vi "Add New XML Tag.vi"(5 "Tag Data":string, 7 "Tag Name":string, 8 "error in (no error)":errorcluster, 10 "Owning Element":refnum<k20>, 11 "XML File Ref in":refnum<k20>) -> (0 "error out":errorcluster, 2 "dup Owning Element":refnum<k20>, 3 "XML File Ref out":refnum<k20>)   [LabVIEW 2020, in "LVLIBP CD XML Updater.lvlib" / "Project XML Editor.lvclass"]
uses:
  Project XML Editor.lvclass
  <vilib>/xml/Close Reference(Node).vi
  <resource>/objmgr/DOMUserDefRef.rc
  <vilib>/xml/NI_XML.lvlib
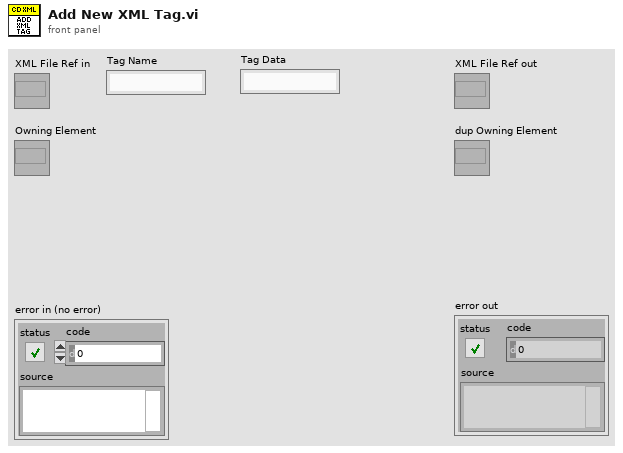
[diagram p1: front panel]
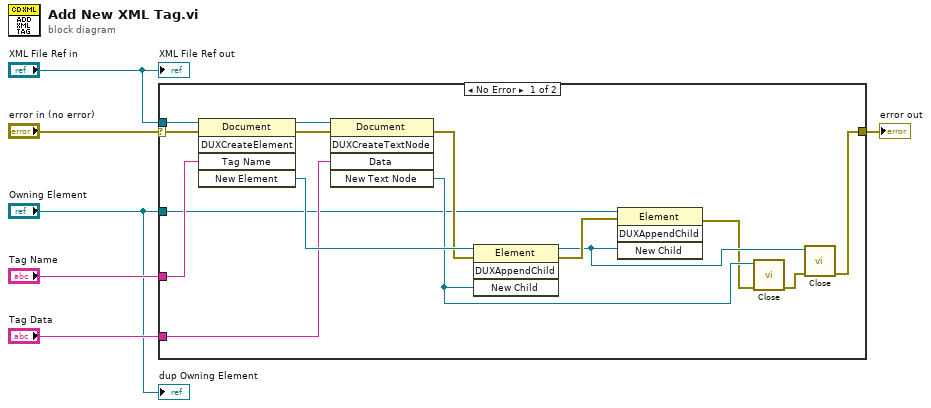
[diagram p0: block diagram]
diagram:
  n1 = case shown="No Error" "error in (no error)" {
    selector: "error in (no error)" -> [w7 w22]
    tunnel: "Tag Name" -> [w12 _]
    tunnel: "Tag Data" -> [w11 _]
    tunnel: "XML File Ref in" -> [w10 _]
    tunnel: "Owning Element" -> [w9 _]
    tunnel: [w8 w22] -> w3
    frame No Error {
      n2 = invoke class="Document" method="DUXCreateElement"(reference=w10, error in=w7, "Tag Name"=w12) -> (reference out=w21:refnum<k20>, error out=w20:errorcluster, "New Element"=w19:refnum<k20>)  [unwired: 2 in, 2 out]
      n3 = invoke class="Document" method="DUXCreateTextNode"(reference=w21, error in=w20, "Data"=w11) -> (error out=w18:errorcluster, "New Text Node"=w14:refnum<k20>)  [unwired: 2 in, 3 out]
      n4 = invoke class="Element" method="DUXAppendChild"(reference=w19, error in=w18, "New Child"=w14) -> (reference out=w15:refnum<k20>, error out=w16:errorcluster)  [unwired: 1 in, 2 out]
      n5 = invoke class="Element" method="DUXAppendChild"(reference=w9, error in=w16, "New Child"=w15) -> (error out=w13:errorcluster)  [unwired: 1 in, 3 out]
      n6 = call-poly <vilib>:"Close.vi"("error in (no error)"=w13, "node"=w14) -> ("error out"=w17:errorcluster)  [unwired: 7 out]
      n7 = call-poly <vilib>:"Close.vi"("error in (no error)"=w17, "node"=w15) -> ("error out"=w8:errorcluster)  [unwired: 7 out]
    }
    frame Error {
    }
  }
  "error out" <- w3
  "XML File Ref out" <- "XML File Ref in"
  "dup Owning Element" <- "Owning Element"
